vi "CloseSensorSession.vi"(8 "error in (no error)":errorcluster, 11 "SiemensDigitalEnergyMeter in":refnum<class "SiemensDigitalEnergyMeter.lvclass">) -> (0 "error out":errorcluster, 3 "SiemensDigitalEnergyMeter out":refnum<class "SiemensDigitalEnergyMeter.lvclass">)   [LabVIEW 2018, in "SensorPlugins.lvlib" / "SiemensDigitalEnergyMeter.lvclass"]
doc: "This VI closes the communicaiton link to the Siemens Digital Energy Meter from the application."
uses:
  SiemensDigitalEnergyMeter.lvclass
  <vilib>/NI/Modbus Library/API/Master/Modbus Master.lvclass
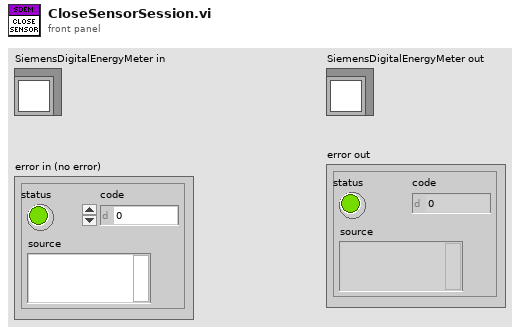
[diagram p1: front panel]
types:
  T1 = typedef "SensorPlugins.lvlib/SiemensDigitalEnergyMeter.lvclass/SiemensDigitalEnergyMeterControls.ctl" = cluster{"Measurement(s)":u16[], "Configuration Commands":string, "Use Measurement Commands Text Box?":bool, "Measurement Commands":string, "Connected?":bool, "Serial Number":string, "IP Address":string, "Port (502)":u16, "Unit ID":u8, "Serial Type":enum16{"RTU", "ASCII"}, "VISA Resource Name":refnum<visa-resource-name>, "Using TCP?":bool}[]
  T2 = typedef "SensorPlugins.lvlib/SiemensDigitalEnergyMeter.lvclass/CommunicationControls.ctl" = refnum<class "Modbus Master.lvclass">[]
  T3 = cluster{"Measurement(s)":u16[], "Configuration Commands":string, "Use Measurement Commands Text Box?":bool, "Measurement Commands":string, "Connected?":bool, "Serial Number":string, "IP Address":string, "Port (502)":u16, "Unit ID":u8, "Serial Type":enum16{"RTU", "ASCII"}, "VISA Resource Name":refnum<visa-resource-name>, "Using TCP?":bool}
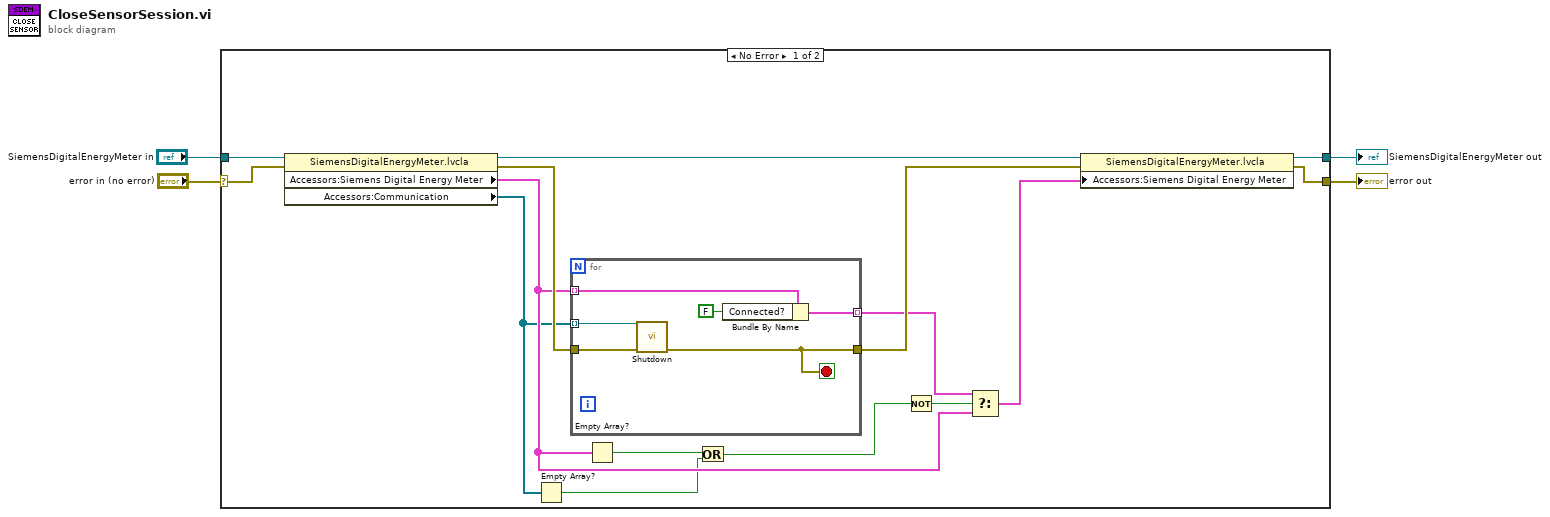
[diagram p0: block diagram]
diagram:
  n1 = case shown="No Error" "error in (no error)" {
    selector: "error in (no error)" -> [w18 w26]
    tunnel: "SiemensDigitalEnergyMeter in" -> [w19 w27]
    tunnel: [w15 w27] -> w2
    tunnel: [w14 w26] -> w1
    frame No Error {
      n2 = property class="SiemensDigitalEnergyMeter.lvcla"(reference=w19, error in=w18) -> (reference out=w16:refnum<class "SiemensDigitalEnergyMeter.lvclass">, error out=w17:errorcluster, "Accessors:Siemens Digital Energy Meter"=w9:T1, "Accessors:Communication"=w8:T2)
      n3 = Empty Array?(array=w8) -> (empty?=w6:bool)
      n4 = for {
        tunnel: w17 -> [w25]
        tunnel: [w24] -> w13
        tunnel: w8 -> [w23] mode=indexing
        tunnel: w9 -> [w22] mode=indexing
        tunnel: [w20] -> w11 mode=indexing
        stop <- w24 stop-if-true
        n5 = call-dynamic "Shutdown.vi"("error in"=w25, "Modbus master in"=w23) -> ("error out"=w24:errorcluster)  [unwired: 9 in]
        n6 = Bundle By Name(cluster=w22, "Connected?"=FALSE) -> (w20:T3)
      }
      n7 = Empty Array?(array=w9) -> (empty?=w7:bool)
      n8 = Or(x=w7, y=w6) -> (x .or. y?=w5:bool)
      n9 = Not(x=w5) -> (.not. x?=w12:bool)
      n10 = Select(t=w11, s=w12, f=w9) -> (s? t:f=w10:T1)
      n11 = property class="SiemensDigitalEnergyMeter.lvcla"(reference=w16, error in=w13, "Accessors:Siemens Digital Energy Meter"=w10) -> (reference out=w15:refnum<class "SiemensDigitalEnergyMeter.lvclass">, error out=w14:errorcluster)
    }
    frame Error {
    }
  }
  "error out" <- w1
  "SiemensDigitalEnergyMeter out" <- w2
